vi "GSM SEND.vi"(11 "Mobile No":string="9540735708") -> ()   [LabVIEW 2013]
uses:
  <vilib>/Instr/_visa.llb/VISA Configure Serial Port (Instr).vi
panel:
  out "AT out Command":string
  in  "VISA resource name":refnum<visa-resource-name>
  in  "Message":string
  out "error out":errorcluster={"status"=TRUE, "code"=-1073807343, "source"="Property Node (arg 1) in VISA Configure Serial Port (Instr).vi->test.vi"}
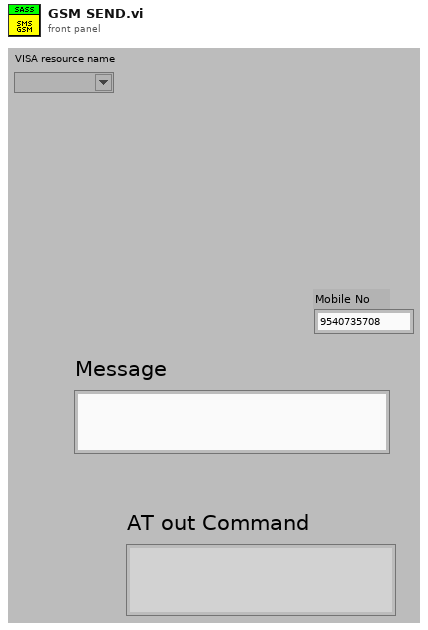
[diagram p1: front panel]
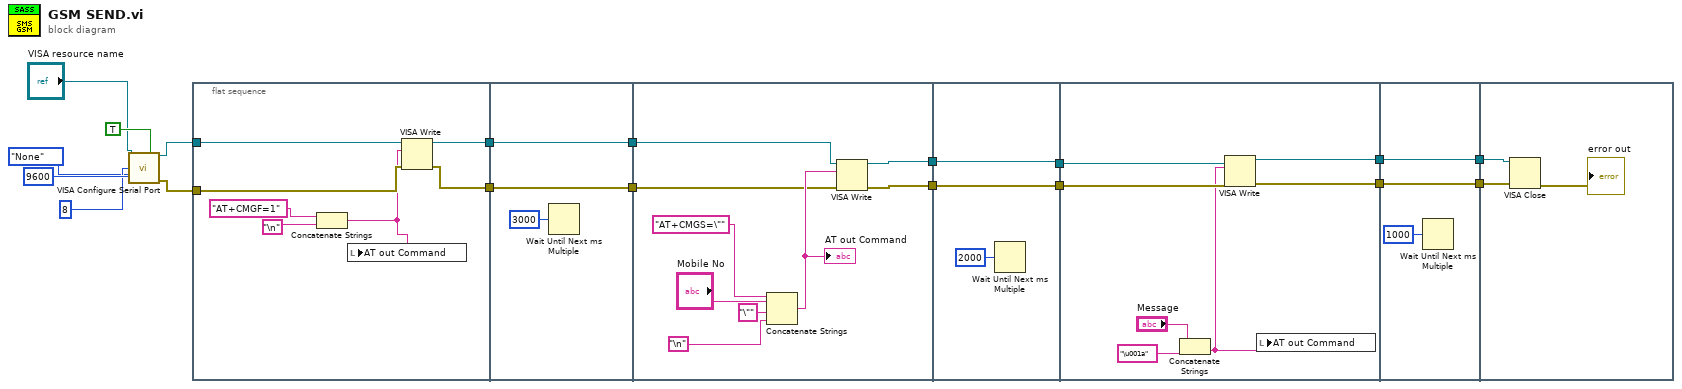
[diagram p0: block diagram]
diagram:
  n1 = call-poly "VISA Configure Serial Port"("VISA resource name"="VISA resource name", "Enable Termination\nChar (T)"=TRUE ("Enable Termination\nChar (T)"), "baud rate (9600)"=u32 9600 ("Baud rate"), "data bits (8)"=u16 8 ("data bits"), "parity (0:none)"=enum16{"None", "Odd", "Even", "Mark", "Space"}."None" ("parity")) -> ("VISA resource name out"=w15:refnum<visa-resource-name>, "error out"=w14:errorcluster)  [unwired: 2 in, 7 out]
  n2 = flat-sequence {
    tunnel: [w24] -> w13
    tunnel: [w23] -> w12
    tunnel: w15 -> [w22]
    tunnel: w14 -> [w21]
    tunnel: [w28] -> w11
    tunnel: w13 -> [w28]
    tunnel: [w27] -> w10
    tunnel: w12 -> [w27]
    tunnel: [w36] -> w9
    tunnel: [w35] -> w8
    tunnel: w11 -> [w34]
    tunnel: w10 -> [w33]
    tunnel: w9 -> [w40]
    tunnel: w8 -> [w39]
    tunnel: [w40] -> w7
    tunnel: [w39] -> w6
    tunnel: w7 -> [w47]
    tunnel: w6 -> [w46]
    tunnel: [w44] -> w5
    tunnel: [w43] -> w4
    tunnel: w5 -> [w51]
    tunnel: [w51] -> w3
    tunnel: w4 -> [w50]
    tunnel: [w50] -> w2
    tunnel: w3 -> [w53]
    tunnel: w2 -> [w52]
    frame #0 {
      n3 = Concatenate Strings("AT+CMGF=1", "\n") -> (w20:string)
      n4 = local write "AT out Command"(w20) -> ()
      n5 = VISA Write(VISA resource name=w22, write buffer=w20, error in (no error)=w21) -> (VISA resource name out=w23:refnum<visa-resource-name>, error out=w24:errorcluster)  [unwired: 1 out]
    }
    frame #1 {
      n6 = Wait Until Next ms Multiple(millisecond multiple=u32 3000) -> ()  [unwired: 1 out]
    }
    frame #2 {
      n7 = Concatenate Strings("AT+CMGS=\"", "Mobile No", "\"" ("string"), "\n") -> (w37:string)
      "AT out Command" <- w37
      n8 = VISA Write(VISA resource name=w33, write buffer=w37, error in (no error)=w34) -> (VISA resource name out=w36:refnum<visa-resource-name>, error out=w35:errorcluster)  [unwired: 1 out]
    }
    frame #3 {
      n9 = Wait Until Next ms Multiple(millisecond multiple=u32 2000) -> ()  [unwired: 1 out]
    }
    frame #4 {
      n10 = Concatenate Strings("Message", "\u001a") -> (w45:string)
      n11 = VISA Write(VISA resource name=w47, write buffer=w45, error in (no error)=w46) -> (VISA resource name out=w43:refnum<visa-resource-name>, error out=w44:errorcluster)  [unwired: 1 out]
      n12 = local write "AT out Command"(w45) -> ()
    }
    frame #5 {
      n13 = Wait Until Next ms Multiple(millisecond multiple=u32 1000) -> ()  [unwired: 1 out]
    }
    frame #6 {
      n14 = VISA Close(VISA resource name=w52, error in (no error)=w53) -> (error out=→"error out":errorcluster)
    }
  }
